vi "close.vi"(8 "error in (no error)":errorcluster, 11 "Relays in":refnum<class "Relays.lvclass">) -> (0 "error out":errorcluster, 3 "Relays out":refnum<class "Relays.lvclass">)   [LabVIEW 2025, in "Relays.lvclass"]
uses:
  Relays.lvclass
  Relays.lvclass/Relays.ctl
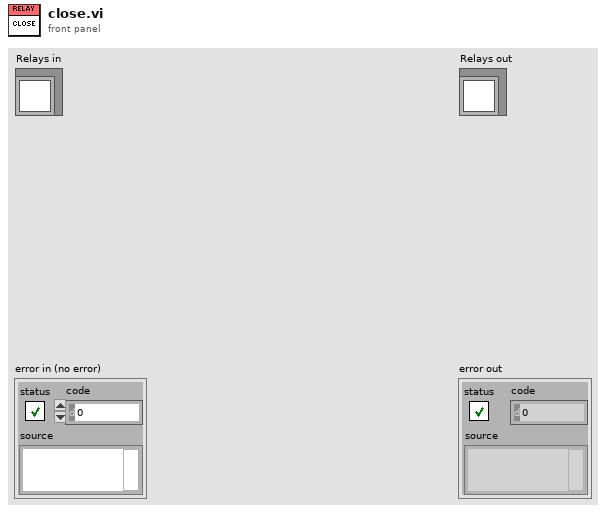
[diagram p1: front panel]
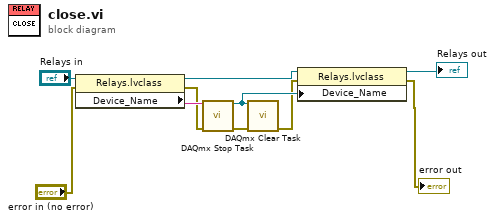
[diagram p0: block diagram]
diagram:
  n1 = property class="Relays.lvclass"(reference="Relays in", error in="error in (no error)") -> (reference out=w4:refnum<class "Relays.lvclass">, error out=w7:errorcluster, "Device_Name"=w8:string)
  n2 = call <vilib>:"DAQmx Stop Task.vi"("task/channels in"=w8, "error in"=w7) -> ("task out"=w5:refnum<k21>, "error out"=w6:errorcluster)  [unwired: 12 in]
  n3 = call <vilib>:"DAQmx Clear Task.vi"("task in"=w5, "error in"=w6) -> ("error out"=w3:errorcluster)  [unwired: 13 in]
  n4 = property class="Relays.lvclass"(reference=w4, error in=w3, "Device_Name"=w5) -> (reference out=→"Relays out":refnum<class "Relays.lvclass">, error out=→"error out":errorcluster)
